vi "Find Speed (Optimized).vi"(0 "[x]":dbl[](array[numeric]), 7 "Speed Settings":T1={"max window"=1400.0, "min window"=45.0, "CommSegments"=2.0}, 13 "index":i32) -> (4 "Speed":dbl)   [LabVIEW 2013]
uses:
  <vilib>/Analysis/2dsp.llb/Power Spectrum (DBL).vi
  <vilib>/Analysis/NI_AALPro.lvlib
panel:
  out "Waveform Graph 2":dbl[][](graph)
  out "Waveform Graph":dbl[][](graph)
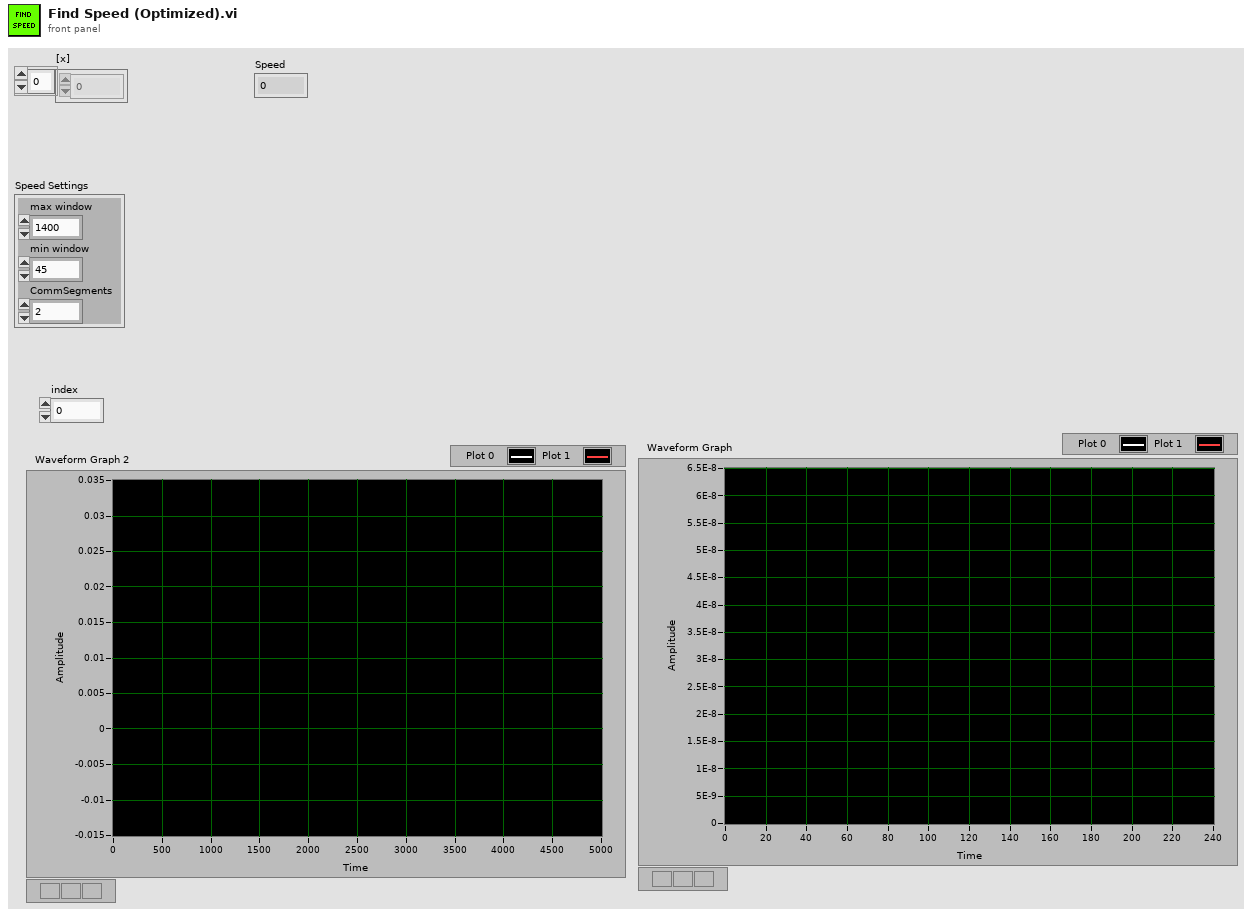
[diagram p1: front panel]
types:
  T1 = cluster{"max window":dbl, "min window":dbl, "CommSegments":dbl}
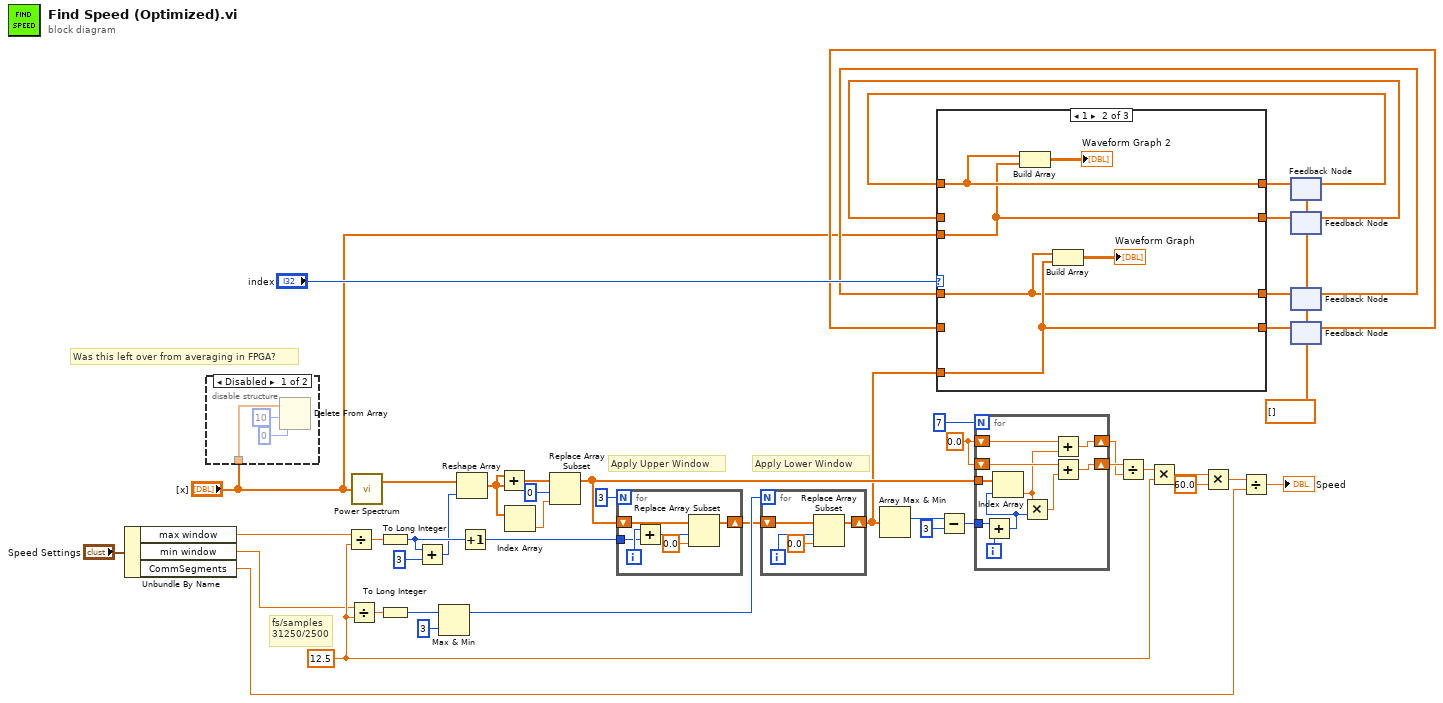
[diagram p0: block diagram]
diagram:
  w10 = dbl[] []
  w43 = 0.0
  w28 = 12.5 ("df")
  # "Was this left over from averaging in FPGA?"
  # "fs/samples\n31250/2500"
  # "Apply Lower Window"
  # "Apply Upper Window"
  n1 = Unbundle By Name("Speed Settings") -> ("max window"=w3:dbl, "min window"=w2:dbl, "CommSegments"=w1:dbl)
  n2 = disable-structure shown="Disabled" {
    disable-tunnel: "[x]" -> [w49 _]
    frame Disabled {
      n3 = Delete From Array(array=w49, length=10, index=0) -> ()  [unwired: 2 out]
    }
    frame Enabled {
    }
  }
  n4 = Divide(x=w3, y=w28) -> (x/y=w26:dbl)
  n5 = Divide(x=w2, y=w28) -> (x/y=w29:dbl)
  n6 = call-poly <vilib>:"Power Spectrum.vi"("X"="[x]") -> ("Power Spectrum"=w17:dbl[])  [unwired: 1 out]
  n7 = To Long Integer(number=w26) -> (32bit integer=w35:i32)
  n8 = To Long Integer(number=w29) -> (32bit integer=w32:i32)
  n9 = Add(x=w35, y=3) -> (x+y=w30:i32)
  n10 = Max & Min(x=w32, y=3) -> (max(x,y)=w38:i32)  [unwired: 1 out]
  n11 = Reshape Array(w17, w30) -> (w25:dbl[])
  n12 = Increment(x=w35) -> (x+1=w36:i32)
  n13 = Add(x=w25, y=w25) -> (x+y=w24:dbl[])
  n14 = Index Array(array=w25) -> (element=w23:dbl)  [unwired: 1 in]
  n15 = Replace Array Subset(array=w24, new element=w23, index=0) -> (w33:dbl[])
  n16 = for {
    N: 3 -> [_]
    shift-right: [w54] -> w37
    shift-left: w33 -> [w55]
    tunnel: w36 -> [w50]
    i -> [w51]
    n17 = Add(x=w51, y=w50) -> (x+y=w53:i32)
    n18 = Replace Array Subset(array=w55, new element=0.0 ("new element/subarray"), index=w53) -> (w54:dbl[])
  }
  n19 = for {
    N: w38 -> [_]
    shift-right: [w58] -> w11
    shift-left: w37 -> [w59]
    i -> [w56]
    n20 = Replace Array Subset(array=w59, new element=0.0 ("new element/subarray"), index=w56) -> (w58:dbl[])
  }
  n21 = Array Max & Min(array=w11) -> (max index (indices)=w39:i32)  [unwired: 3 out]
  n22 = Subtract(x=w39, y=3) -> (x-y=w42:i32)
  n23 = for {
    N: 7 ("span") -> [_]
    tunnel: w42 -> [w69]
    tunnel: w33 -> [w68]
    shift-right: [w64] -> w44
    shift-left: w43 -> [w65]
    shift-right: [w62] -> w45
    shift-left: w43 -> [w63]
    i -> [w67]
    n24 = Add(x=w69, y=w67) -> (x+y=w66:i32)
    n25 = Index Array(array=w68, index=w66) -> (element=w60:dbl)
    n26 = Multiply(x=w60, y=w66) -> (x*y=w61:dbl)
    n27 = Add(x=w65, y=w60) -> (x+y=w64:dbl)
    n28 = Add(x=w63, y=w61) -> (x+y=w62:dbl)
  }
  n29 = Divide(x=w45, y=w44) -> (x/y=w46:dbl)
  n30 = Multiply(x=w46, y=w28) -> (x*y=w21:dbl)
  n31 = Multiply(x=w21, y=60.0) -> (x*y=w20:dbl)
  n32 = Divide(x=w20, y=w1) -> (x/y=→"Speed":dbl)
  n33 = feedback #1(w10) -> (w6:dbl[])
  n34 = feedback #2(w10) -> (w7:dbl[])
  n35 = feedback #3(w10) -> (w13:dbl[])
  n36 = feedback #4(w10) -> (w12:dbl[])
  n37 = case shown="1" "index" {
    tunnel: w12 -> [w72 _ w83]
    tunnel: [w72 w79 w83] -> w15
    tunnel: [w73 w78 w82] -> w14
    tunnel: w13 -> [_ w78 w82]
    tunnel: w11 -> [w73 w79 _]
    tunnel: [w71 w76 w81] -> w9
    tunnel: [w70 w75 w80] -> w8
    tunnel: w7 -> [w70 _ w80]
    tunnel: w6 -> [_ w76 w81]
    tunnel: "[x]" -> [w71 w75 _]
    frame 0 {
    }
    frame 1 {
      n38 = Build Array(w76, w75) -> (→"Waveform Graph 2":dbl[][])
      n39 = Build Array(w78, w79) -> (→"Waveform Graph":dbl[][])
    }
    frame Default {
    }
  }
  n40 = feedback-in #1(w9) -> ()
  n41 = feedback-in #2(w8) -> ()
  n42 = feedback-in #3(w14) -> ()
  n43 = feedback-in #4(w15) -> ()
